vi "VG_VCellMin30.vi"() -> ()   [LabVIEW 2020]
panel:
  out "VCellMin30":dbl
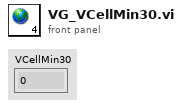
[diagram p1: front panel]
diagram:
